vi "nPoints Concept - Microphone.vi"() -> ()   [LabVIEW 2013]
uses:
  <vilib>/DAQmx/read.llb/DAQmx Read (Analog Wfm 1Chan NSamp).vi
  <vilib>/DAQmx/create/channels.llb/DAQmx Create Channel (AI-Voltage-Basic).vi
  <vilib>/DAQmx/configure/timing.llb/DAQmx Timing (Sample Clock).vi
  <vilib>/DAQmx/miscellaneous.llb/DAQmx Fill In Error Info.vi
  <vilib>/ptbypt/NI_PtbyPt.lvlib
panel:
  in  "Stop":bool
  out "Waveform Chart":waveform(dbl)(graph)
  in  "Samples to Avg":i32=10
  in  "y":dbl=200.0
  out "VU Meter R":dbl(knob) scale=0.0..12.0
  # "Microphone"
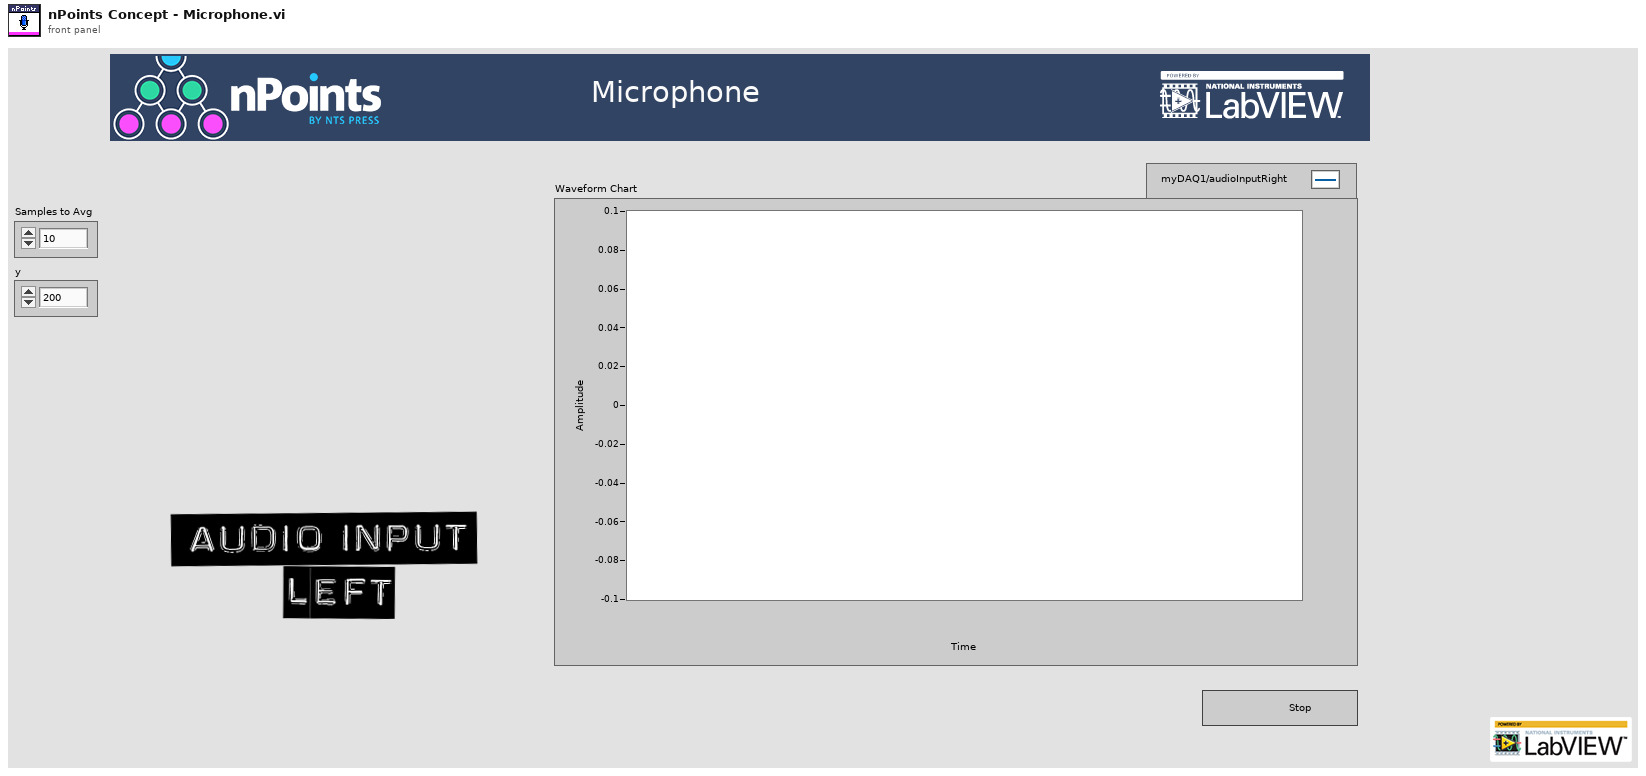
[diagram p1: front panel]
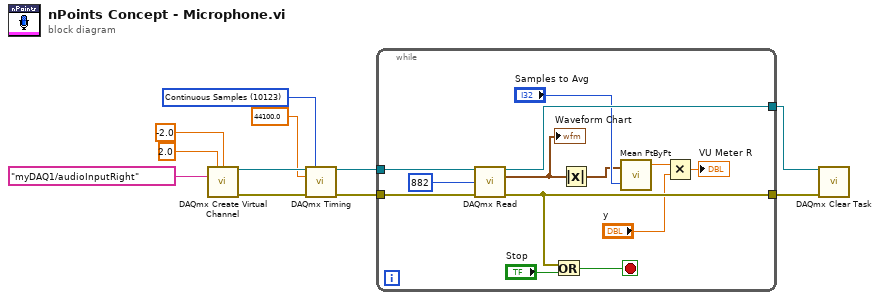
[diagram p0: block diagram]
diagram:
  w2 = 10123 items=["Finite Samples"=10178, "Continuous Samples"=10123, "Hardware Timed Single Point"=12522] ("sample mode")
  n1 = call-poly <vilib>:"DAQmx Create Virtual Channel.vi"("maximum value"=2.0, "minimum value"=-2.0, "physical channels"=tag "myDAQ1/audioInputRight") -> ("task out"=w11:refnum<k21>, "error out"=w10:errorcluster)  [unwired: 11 in]
  n2 = call-poly <vilib>:"DAQmx Timing.vi"("task/channels in"=w11, "sample mode"=w2, "rate"=44100.0, "error in"=w10) -> ("task out"=w8:refnum<k21>, "error out"=w9:errorcluster)  [unwired: 10 in]
  n3 = while {
    tunnel: w9 -> [w24]
    tunnel: w8 -> [w23]
    tunnel: [w22] -> w7
    tunnel: [w19] -> w6
    stop <- w20 stop-if-true
    n4 = call-poly <vilib>:"DAQmx Read.vi"("task/channels in"=w23, "number of samples per channel"=882, "error in"=w24) -> ("task out"=w22:refnum<k21>, "data"=w16:waveform(dbl), "error out"=w19:errorcluster)  [unwired: 10 in]
    "Waveform Chart" <- w16
    n5 = Or(x=w19, y="Stop") -> (x .or. y?=w20:bool)
    n6 = Absolute Value(x=w16) -> (abs(x)=w15:waveform(dbl))
    n7 = call <vilib>:"Mean PtByPt.vi"("x"=w15, "sample length"="Samples to Avg") -> ("mean"=w14:dbl)  [unwired: 2 in, 1 out]
    n8 = Multiply(x=w14, y="y") -> (x*y=→"VU Meter R":dbl)
  }
  n9 = call <vilib>:"DAQmx Clear Task.vi"("task in"=w7, "error in"=w6) -> ()  [unwired: 13 in, 1 out]
